vi "LV6_1.vi"() -> ()   [LabVIEW 2011]
uses:
  <vilib>/sound2/lvsound2.llb/Sampling Mode.ctl
  <vilib>/Utility/file.llb/Read From Spreadsheet File (DBL).vi
  <vilib>/imath/engines/lvmath2/RunTimeEngine/ErrorHandling/NIMS_Finalize Error.vi
  <vilib>/imath/engines/lvmath2/RunTimeEngine/BuiltInFunctions/length/NIMS_length(GV).vi
  <instcachedir>/0/NIMS_length(GV)_08A3D13377FD4E4B96F5795FBF3698FA.lvgen/NIMS_length(GV)_08A3D13377FD4E4B96F5795FBF3698FA_000.vi
  <vilib>/imath/engines/lvmath2/RunTimeEngine/NodeEndStatement/NIMS_NodeEndStatement_Output.vi
  <instcachedir>/0/NIMS_NodeEndStatement_Output_53EC0D466D134D7ABD903AC30B43404B.lvgen/NIMS_NodeEndStatement_Output_53EC0D466D134D7ABD903AC30B43404B_000.vi
  <instcachedir>/0/NIMS_NodeEndStatement_Output_53EC0D466D134D7ABD903AC30B43404B.lvgen/NIMS_NodeEndStatement_Output_53EC0D466D134D7ABD903AC30B43404B_005.vi
  <instcachedir>/0/NIMS_NodeEndStatement_Output_53EC0D466D134D7ABD903AC30B43404B.lvgen/NIMS_NodeEndStatement_Output_53EC0D466D134D7ABD903AC30B43404B_009.vi
  <vilib>/imath/engines/lvmath2/RunTimeEngine/RangeToken/NIMS_Range.vi
  <instcachedir>/0/NIMS_Range_0B7635FB69F84E19AA68E7FF959DF37C.lvgen/NIMS_Range_0B7635FB69F84E19AA68E7FF959DF37C_000.vi
  <vilib>/imathl/engines/lvmath/Functions/Error Handling/Create Error.vi
  <vilib>/imath/engines/lvmath2/RunTimeEngine/ArithmeticOperatorToken/NIMS_ArithmeticOperator_plus.vi
  <instcachedir>/0/NIMS_ArithmeticOperator_plus_1E95F7DAB906458CBECCADBE8E6FD739.lvgen/NIMS_ArithmeticOperator_plus_1E95F7DAB906458CBECCADBE8E6FD739_004.vi
  <vilib>/imath/engines/lvmath2/RunTimeEngine/BuiltInFunctions/cos/NIMS_cos(C).vi
  <instcachedir>/0/NIMS_cos(C)_A49CF571DB584453A51052084B12F0F9.lvgen/NIMS_cos(C)_A49CF571DB584453A51052084B12F0F9_001.vi
  <vilib>/imath/engines/lvmath2/RunTimeEngine/ArithmeticOperatorToken/NIMS_ArithmeticOperator_times.vi
  <instcachedir>/0/NIMS_ArithmeticOperator_times_3FA9DDB491BD45F6905798C0465C9825.lvgen/NIMS_ArithmeticOperator_times_3FA9DDB491BD45F6905798C0465C9825_003.vi
  <vilib>/imath/engines/lvmath2/RunTimeEngine/BuiltInFunctions/fft/NIMS_fft(GV).vi
  <instcachedir>/0/NIMS_fft(GV)_4C6467FC22F84E4BA42517A07EF978B0.lvgen/NIMS_fft(GV)_4C6467FC22F84E4BA42517A07EF978B0_000.vi
  <vilib>/imath/engines/lvmath2/RunTimeEngine/ErrorHandling/NIMS_Error From Error Code.vi
  <instcachedir>/0/NIMS_fft(GV)_4C6467FC22F84E4BA42517A07EF978B0.lvgen/NIMS_fft(GV)_4C6467FC22F84E4BA42517A07EF978B0_001.vi
  <vilib>/imath/engines/lvmath2/RunTimeEngine/BuiltInFunctions/ifft/NIMS_ifft(CV).vi
  <vilib>/imath/engines/lvmath2/RunTimeEngine/ErrorHandling/NIMS_Create Error From Enums.vi
  <vilib>/imath/engines/lvmath2/RunTimeEngine/VariableToken/Read/NIMS_Get Elements - RV(_) - Check.vi
  <instcachedir>/0/NIMS_Get Elements - RV(_) - Check_B511B9D8E05044FE80F9F088FE24B20C.lvgen/NIMS_Get Elements - RV(_) - Check_B511B9D8E05044FE80F9F088FE24B20C_003.vi
  <vilib>/imath/engines/lvmath2/RunTimeEngine/BuiltInFunctions/abs/NIMS_abs(signed).vi
  <instcachedir>/0/NIMS_abs(signed)_C4FCB8E6058B49B797C7C8D53CA5F6EC.lvgen/NIMS_abs(signed)_C4FCB8E6058B49B797C7C8D53CA5F6EC_006.vi
  <vilib>/sound2/lvsound2.llb/Sound Output Write (DBL Single).vi
panel:
  in  "notch frequency":dbl(slide)=800.0 scale=600.0..2000.0
  in  "minus real part of poles":dbl(slide)=100.0 scale=10.0..500.0
  in  "Interference frequency":dbl(slide)=800.0 scale=600.0..2000.0
  in  "Interference level":dbl(slide)=1.0 scale=0.0..1.0
  out "Filter impulse (time domain)":cluster{"t":dbl[], "Y":dbl[]}(graph)
  out "Signal + interference (freq domain)":cluster{"F":dbl[], "FYI":dbl[]}(graph)
  out "Signal + interference (time domain)":cluster{"t":dbl[], "Y":dbl[]}(graph)
  out "Filtered signal (freq domain)":cluster{"F":dbl[], "FZI":dbl[]}[](graph)
  out "Original signal (freq domain)":cluster{"F":dbl[], "FXI":dbl[]}(graph)
  out "Original signal (time domain)":cluster{"t":dbl[], "first row":dbl[]}(graph)
  out "Filtered signal (time domain)":cluster{"t":dbl[], "Y":dbl[]}(graph)
  in  "Play original sound":bool
  in  "Play noisy sound":bool
  in  "Play filtered sound":bool
  in  "stop":bool
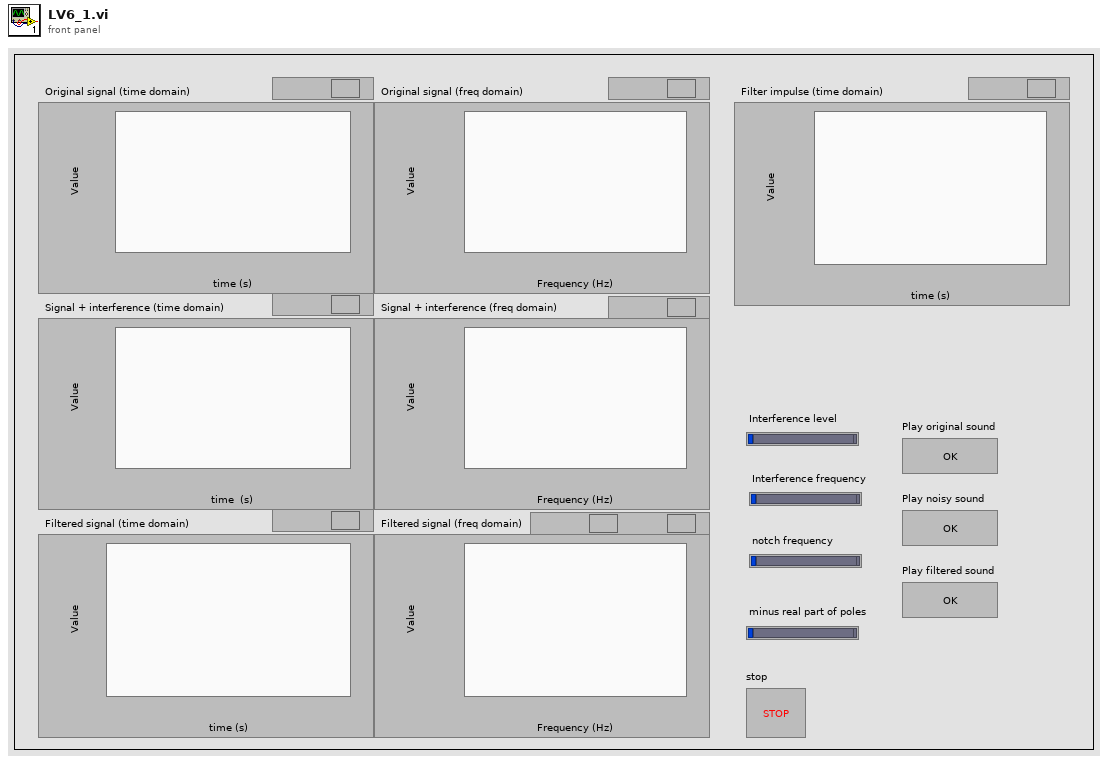
[diagram p1: front panel]
types:
  T1 = typedef "Sampling Mode.ctl" = i32
  T2 = typedef "Sound Output Task ID.ctl" = u32
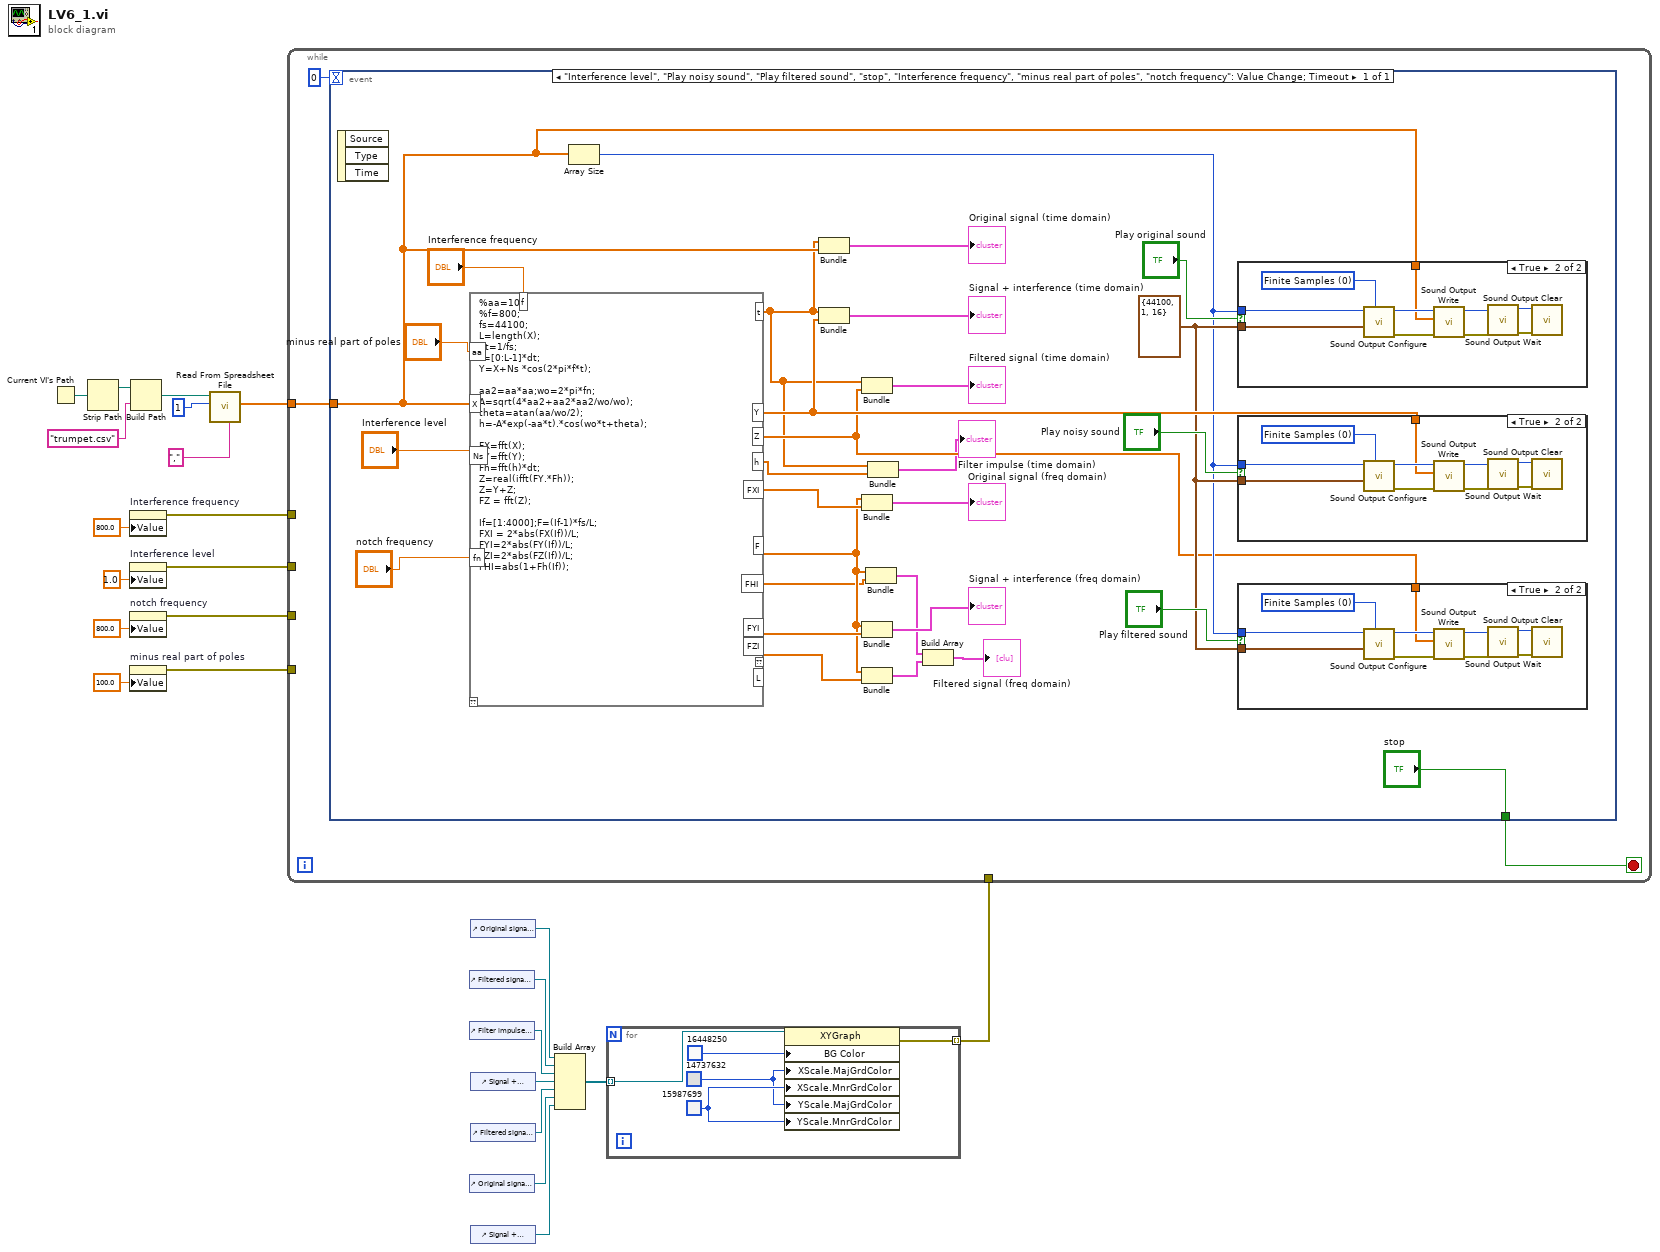
[diagram p0: block diagram]
diagram:
  n1 = Current VI's Path() -> (path=w24:path)
  n2 = Strip Path(path=w24) -> (stripped path=w23:path)  [unwired: 1 out]
  n3 = property on="Interference frequency" class="Slide (strict)"("Value"=800.0 ("Interference frequency")) -> (error out=w17:errorcluster)  [unwired: 2 in, 1 out]
  n4 = property on="Interference level" class="Slide (strict)"("Value"=1.0 ("Interference level")) -> (error out=w16:errorcluster)  [unwired: 2 in, 1 out]
  n5 = property on="notch frequency" class="Slide (strict)"("Value"=800.0 ("notch frequency")) -> (error out=w15:errorcluster)  [unwired: 2 in, 1 out]
  n6 = property on="minus real part of poles" class="Slide (strict)"("Value"=100.0 ("minus real part of poles")) -> (error out=w14:errorcluster)  [unwired: 2 in, 1 out]
  n7 = Build Path(base path=w23, name or relative path="trumpet.csv") -> (appended path=w21:path)
  n8 = call-poly <vilib>:"Read From Spreadsheet File.vi"("delimiter (\\t)"="," ("delimiter (\\t)"), "number of rows (all:-1)"=1, "file path (dialog if empty)"=w21) -> ("first row"=w18:dbl[])  [unwired: 4 in, 4 out]
  n9 = control-ref of="Filtered signal (time domain)"() -> (w8:refnum<vi>)
  n10 = control-ref of="Filter impulse (time domain)"() -> (w7:refnum<vi>)
  n11 = control-ref of="Original signal (freq domain)"() -> (w4:refnum<vi>)
  n12 = control-ref of="Original signal (time domain)"() -> (w9:refnum<vi>)
  n13 = control-ref of="Signal + interference (time domain)"() -> (w6:refnum<vi>)
  n14 = control-ref of="Filtered signal (freq domain)"() -> (w5:refnum<vi>)
  n15 = control-ref of="Signal + interference (freq domain)"() -> (w3:refnum<vi>)
  n16 = Build Array(w9, w8, w7, w6, w5, w4, w3) -> (w2:refnum<vi>[])
  n17 = for {
    tunnel: w2 -> [w26] mode=indexing
    tunnel: [w25] -> w1 mode=indexing
    w28 = u32 15987699
    w27 = u32 14737632
    n18 = property class="XYGraph"(reference=w26, "BG Color"=u32 16448250, "XScale.MajGrdColor"=w27, "XScale.MnrGrdColor"=w28, "YScale.MajGrdColor"=w27, "YScale.MnrGrdColor"=w28) -> (error out=w25:errorcluster)  [unwired: 1 in, 1 out]
  }
  n19 = while {
    tunnel: w18 -> [w32]
    tunnel: w17 -> [_]
    tunnel: w16 -> [_]
    tunnel: w15 -> [_]
    tunnel: w14 -> [_]
    tunnel: w1 -> [_]
    stop <- w31 stop-if-true
    n20 = event shown="[0] \"Interference level\", \"Play noisy sound\", \"Play filtered sound\", \"stop\", \"Interference frequency\", \"minus real part of poles\", \"notch frequency\": Value Change;  Timeout" {
      selector: _ -> [_]
      dyn-events: _ -> [_]
      timeout: 0 -> [_]
      tunnel: w32 -> [w56]
      tunnel: ["stop"] -> w31
      event "Interference level", "Play noisy sound", "Play filtered sound", "stop", "Interference frequency", "minus real part of poles", "notch frequency": Value Change; Timeout {
        w52 = cluster{"fs":i32, i32, i32} {"fs"=44100, 1, 16}
        n21 = event-data() -> ()  [unwired: 1 in, 3 out]
        n22 = mathscript code="%aa=100;\n%f=800;\nfs=44100;\nL=length(X);\ndt=1/fs;\nt=[0:L-1]*dt;\nY=X+Ns *cos(2*pi*f*t);\n\naa2=aa*aa;wo=2*pi*fn;\nA=sqrt(4*aa2+aa2*aa2/wo/wo);\ntheta=atan(aa/wo/2);\nh=-A*exp(-aa*t).*cos(wo*t+theta);\n\nFX=fft(X);\nFY=fft(Y);\nFh=fft(h)*dt;\nZ=real(ifft(FY.*Fh));\nZ=Y+Z;\nFZ = fft(Z);\n\nIf=[1:4000];F=(If-1)*fs/L;\nFXI = 2*abs(FX(If))/L;\nFYI=2*abs(FY(If))/L;\nFZI=2*abs(FZ(If))/L;\nFHI=abs(1+Fh(If));"("X"=w56, "aa"="minus real part of poles", "Ns"="Interference level", "f"="Interference frequency", "fn"="notch frequency") -> ("Z"=w50:dbl[], "Y"=w54:dbl[], "F"=w45:dbl[], "FYI"=w48:dbl[], "t"=w39:dbl[], "FZI"=w46:dbl[], "FXI"=w47:dbl[], "FHI"=w41:dbl[], "h"=w38:cdb[])  [unwired: 1 in, 2 out]
        n23 = Array Size(array=w56) -> (size(s)=w51:i32)
        n24 = Bundle("t"=w39, "first row"=w56) -> (→"Original signal (time domain)":cluster{"t":dbl[], "first row":dbl[]})  [unwired: 1 in]
        n25 = Bundle("t"=w39, "Y"=w54) -> (→"Signal + interference (time domain)":cluster{"t":dbl[], "Y":dbl[]})  [unwired: 1 in]
        n26 = Bundle("t"=w39, "Z"=w50) -> (→"Filtered signal (time domain)":cluster{"t":dbl[], "Z":dbl[]})  [unwired: 1 in]
        n27 = Bundle("F"=w45, "FXI"=w47) -> (→"Original signal (freq domain)":cluster{"F":dbl[], "FXI":dbl[]})  [unwired: 1 in]
        n28 = Bundle("F"=w45, "FYI"=w48) -> (→"Signal + interference (freq domain)":cluster{"F":dbl[], "FYI":dbl[]})  [unwired: 1 in]
        n29 = Bundle("F"=w45, "FZI"=w46) -> (w35:cluster{"F":dbl[], "FZI":dbl[]})  [unwired: 1 in]
        n30 = Bundle("F"=w45, "FHI"=w41) -> (w36:cluster{"F":dbl[], "FHI":dbl[]})  [unwired: 1 in]
        n31 = Bundle("t"=w39, "h"=w38) -> (→"Filter impulse (time domain)":cluster{"t":dbl[], "h":cdb[]})  [unwired: 1 in]
        n32 = Build Array(w36, w35) -> (→"Filtered signal (freq domain)":cluster{"F":dbl[], "FZI":dbl[]}[])
        n33 = case shown="True" "Play original sound" {
          tunnel: w52 -> [_ w389]
          tunnel: w51 -> [_ w387]
          tunnel: w56 -> [_ w386]
          frame False {
          }
          frame True {
            w388 = T1 0 items=["Finite Samples", "Continuous Samples"] ("sample mode")
            n34 = call <vilib>:"Sound Output Configure.vi"("number of samples/ch"=w387, "sample mode"=w388, "sound format"=w389) -> ("error out"=w390:errorcluster, "task ID"=w395:T2)  [unwired: 7 in]
            n35 = call-poly <vilib>:"Sound Output Write.vi"("error in (no error)"=w390, "data"=w386, "task ID"=w395) -> ("error out"=w391:errorcluster, "task ID out"=w392:T2)  [unwired: 7 in]
            n36 = call <vilib>:"Sound Output Wait.vi"("error in (no error)"=w391, "task ID"=w392) -> ("error out"=w394:errorcluster, "task ID out"=w393:T2)  [unwired: 8 in]
            n37 = call <vilib>:"Sound Output Clear.vi"("error in (no error)"=w394, "task ID"=w393) -> ()  [unwired: 9 in, 1 out]
          }
        }
        n38 = case shown="True" "Play noisy sound" {
          tunnel: w52 -> [_ w379]
          tunnel: w51 -> [_ w377]
          tunnel: w54 -> [_ w376]
          frame False {
          }
          frame True {
            w378 = T1 0 items=["Finite Samples", "Continuous Samples"] ("sample mode")
            n39 = call <vilib>:"Sound Output Configure.vi"("number of samples/ch"=w377, "sample mode"=w378, "sound format"=w379) -> ("error out"=w380:errorcluster, "task ID"=w385:T2)  [unwired: 7 in]
            n40 = call-poly <vilib>:"Sound Output Write.vi"("error in (no error)"=w380, "data"=w376, "task ID"=w385) -> ("error out"=w381:errorcluster, "task ID out"=w382:T2)  [unwired: 7 in]
            n41 = call <vilib>:"Sound Output Wait.vi"("error in (no error)"=w381, "task ID"=w382) -> ("error out"=w384:errorcluster, "task ID out"=w383:T2)  [unwired: 8 in]
            n42 = call <vilib>:"Sound Output Clear.vi"("error in (no error)"=w384, "task ID"=w383) -> ()  [unwired: 9 in, 1 out]
          }
        }
        n43 = case shown="True" "Play filtered sound" {
          tunnel: w52 -> [_ w369]
          tunnel: w51 -> [_ w367]
          tunnel: w50 -> [_ w366]
          frame False {
          }
          frame True {
            w368 = T1 0 items=["Finite Samples", "Continuous Samples"] ("sample mode")
            n44 = call <vilib>:"Sound Output Configure.vi"("number of samples/ch"=w367, "sample mode"=w368, "sound format"=w369) -> ("error out"=w370:errorcluster, "task ID"=w375:T2)  [unwired: 7 in]
            n45 = call-poly <vilib>:"Sound Output Write.vi"("error in (no error)"=w370, "data"=w366, "task ID"=w375) -> ("error out"=w371:errorcluster, "task ID out"=w372:T2)  [unwired: 7 in]
            n46 = call <vilib>:"Sound Output Wait.vi"("error in (no error)"=w371, "task ID"=w372) -> ("error out"=w374:errorcluster, "task ID out"=w373:T2)  [unwired: 8 in]
            n47 = call <vilib>:"Sound Output Clear.vi"("error in (no error)"=w374, "task ID"=w373) -> ()  [unwired: 9 in, 1 out]
          }
        }
      }
    }
  }
